vi "GET_issue_by_id.vi"(8 "error in (no error)":errorcluster, 10 "issue id":i32, 11 "REST Client in":refnum<class "REST Client.lvclass">) -> (0 "error out":errorcluster, 2 "local_issue":T1, 3 "REST Client out":refnum<class "REST Client.lvclass">)   [LabVIEW 2024]
uses:
  <vilib>/addons/_JKI.lib/REST Client/classes/REST Client/REST Client.lvclass
  definitions/local_issue.ctl
  definitions/comicvine_issue.generic_credit.ctl
  definitions/comicvine_issue.associated_image.ctl
  definitions/comicvine_issue.person_credit.ctl
  <vilib>/addons/_JKI.lib/REST Client/classes/REST Client/HTTP Header.ctl
  <vilib>/NI/Advanced HTTP Client/Header--Combo Box.ctl
  definitions/comicvine_issue.ctl
  definitions/comicvine_issue.results.ctl
  <vilib>/NI/Advanced HTTP Client/Session.lvclass
  <userlib>/_OpenG.lib/string/string.llb/openg_string.lvlib
  <vilib>/addons/_JKI.lib/Serialization/JSON/JKI JSON Serialization.lvlib
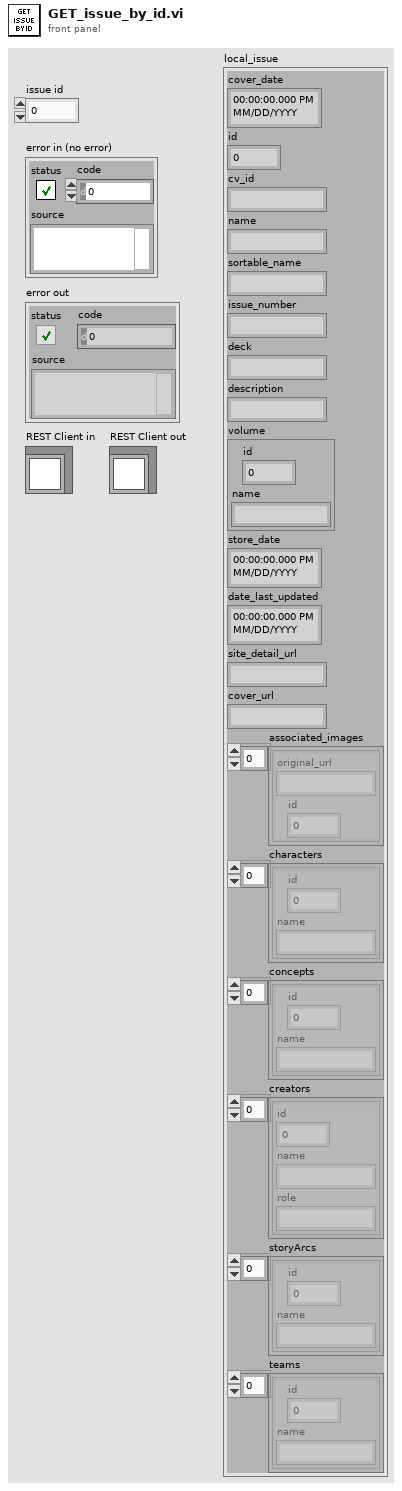
[diagram p1: front panel]
types:
  T1 = typedef "local_issue.ctl" = cluster{"cover_date":timestamp, "id":i32, "cv_id":string, "name":string, "sortable_name":string, "issue_number":string, "deck":string, "description":string, "volume":T2, "store_date":timestamp, "date_last_updated":timestamp, "site_detail_url":string, "cover_url":string, "associated_images":T3[], "characters":T2[], "concepts":T2[], "creators":T4[], "storyArcs":T2[], "teams":T2[]}
  T2 = typedef "comicvine_issue.generic_credit.ctl" = cluster{"id":i32, "name":string}
  T3 = typedef "comicvine_issue.associated_image.ctl" = cluster{"original_url":string, "id":i32}
  T4 = typedef "comicvine_issue.person_credit.ctl" = cluster{"id":i32, "name":string, "role":string}
  T5 = typedef "comicvine_issue.ctl" = cluster{"error":string, "limit":i32, "offset":i32, "number_of_page_results":i32, "number_of_total_results":i32, "status_code":i32, "results":T6}
  T6 = typedef "comicvine_issue.results.ctl" = cluster{"associated_images":T3[], "character_credits":T2[], "concept_credits":T2[], "cover_date":timestamp, "date_last_updated":timestamp, "deck":string, "description":string, "id":i32, "image":cluster{"original_url":string}, "issue_number":string, "name":string, "person_credits":T4[], "site_detail_url":string, "store_date":timestamp, "story_arc_credits":T2[], "team_credits":T2[], "volume":T2}
  T7 = typedef "REST Client.lvlib/REST Client.lvclass/HTTP Header.ctl" = cluster{"header":T8, "value":string}
  T8 = typedef "lib_NI_Advanced HTTP Client.lvlib/Session.lvclass/Header--Combo Box.ctl" = string
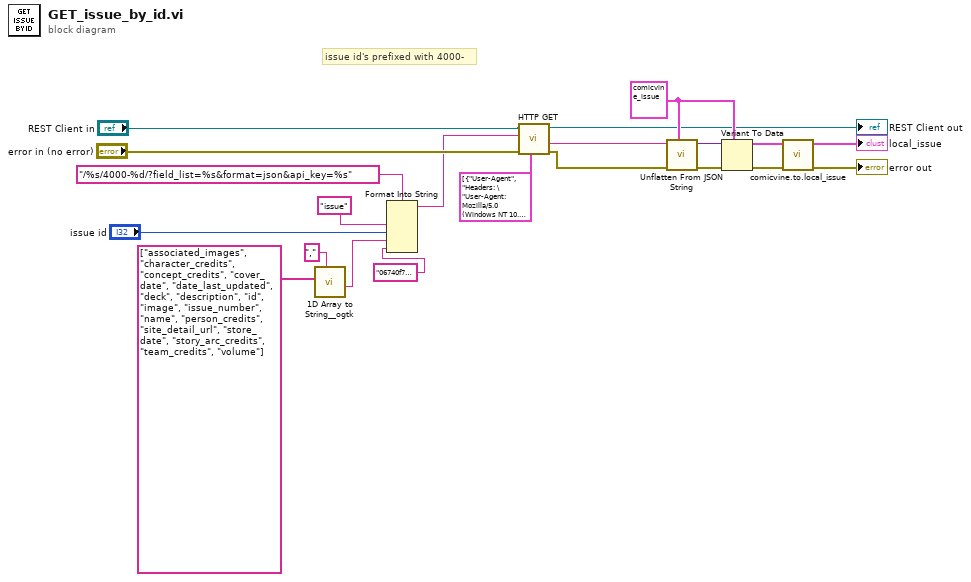
[diagram p0: block diagram]
diagram:
  w7 = T5 {"error"="", "limit"=0, "offset"=0, "number_of_page_results"=0, "number_of_total_results"=0, "status_code"=0, "results"={"associated_images"=[], "character_credits"=[], "concept_credits"=[], "cover_date"=timestamp(0 s since 1904-01-01), "date_last_updated"=timestamp(0 s since 1904-01-01), "deck"="", "description"="", "id"=0, "image"={"original_url"=""}, "issue_number"="", "name"="", "person_credits"=[], "site_detail_url"="", "store_date"=timestamp(0 s since 1904-01-01), "story_arc_credits"=[], "team_credits"=[], "volume"={"id"=0, "name"=""}}} ("issue")
  # "issue id's prefixed with 4000-"
  n1 = call <userlib>:"1D Array to String__ogtk.vi"("delimiter (Tab)"=",", "Array of Strings"=string[] ["associated_images", "character_credits", "concept_credits", "cover_date", "date_last_updated", "deck", "description", "id", "image", "issue_number", "name", "person_credits", "site_detail_url", "store_date", "story_arc_credits", "team_credits", "volume"]) -> ("delimited string"=w11:string)  [unwired: 9 in]
  n2 = Format Into String(format string="/%s/4000-%d/?field_list=%s&format=json&api_key=%s", "issue" ("resource"), "issue id", w11, "06740f73403e0b211d597c50ea94c7f16ea5e8ea") -> (resulting string=w16:string)  [unwired: 2 in, 1 out]
  n3 = call-dynamic "HTTP GET.vi"("request specific headers"=T7[] [{"header"="User-Agent", "value"="Headers: \"User-Agent: Mozilla/5.0 (Windows NT 10.0; Win64; x64) AppleWebKit/537.36 (KHTML, like Gecko) Chrome/91.0.4472.101 Safari/537.36\""}], "error in (no error)"="error in (no error)", "Path"=w16, "REST Client in"="REST Client in") -> ("error out"=w21:errorcluster, "Response body"=w10:string, "REST Client out"=→"REST Client out":refnum<class "REST Client.lvclass">)  [unwired: 2 in, 3 out]
  n4 = call <vilib>:"Unflatten From JSON String.vi"("Type and Defaults"=w7, "error in"=w21, "JSON String"=w10) -> ("error out"=w9:errorcluster, "Variant"=w8:variant)  [unwired: 7 in]
  n5 = Variant To Data(error in=w9, type=w7, Variant=w8) -> (data=w4:T5, error out=w3:errorcluster)
  n6 = call "comicvine.to.local_issue.vi"("error in (no error)"=w3, "cv_issue"=w4) -> ("error out"=→"error out":errorcluster, "local_issue"=→"local_issue":T1)  [unwired: 8 in]
